vi "Configure Measurement Source.vi"(6 "Measurement Source 2 (0: Channel 1)":i32(ring) items=["Channel 1", "Channel 2", "Channel 3", "Channel 4", "Function 1", "Function 2", "Function 3", "Function 4", "Digital 0", "Digital 1", "Digital 2", "Digital 3", "Digital 4", "Digital 5", "Digital 6", "Digital 7", "Digital 8", "Digital 9", "Digital 10", "Digital 11", "Digital 12", "Digital 13", "Digital 14", "Digital 15", "Memory 1", "Memory 2", "Memory 3", "Memory 4", "Clock", "MTrend", "MSpectrum", "Equalized"], 8 "error in (no error)":errorcluster, 9 "Measurement Source 1 (0: Channel 1)":i32(ring) items=["Channel 1", "Channel 2", "Channel 3", "Channel 4", "Function 1", "Function 2", "Function 3", "Function 4", "Digital 0", "Digital 1", "Digital 2", "Digital 3", "Digital 4", "Digital 5", "Digital 6", "Digital 7", "Digital 8", "Digital 9", "Digital 10", "Digital 11", "Digital 12", "Digital 13", "Digital 14", "Digital 15", "Memory 1", "Memory 2", "Memory 3", "Memory 4", "Clock", "MTrend", "MSpectrum", "Equalized"], 10 "Source Count (0: 1 Source)":u16(ring) items=["1 Source", "2 Source"], 11 "VISA resource name":refnum<visa-resource-name>) -> (0 "error out":errorcluster, 3 "VISA resource name out":refnum<visa-resource-name>)   [LabVIEW 2020, in "Agilent 90000 Series.lvlib"]
doc: "Configures the source for measurements. You can specify one or two sources with this command. Most measurements are made on the first specified source. The delta time measurement uses two sources if two are specified."
uses:
  Agilent 90000 Series.lvlib
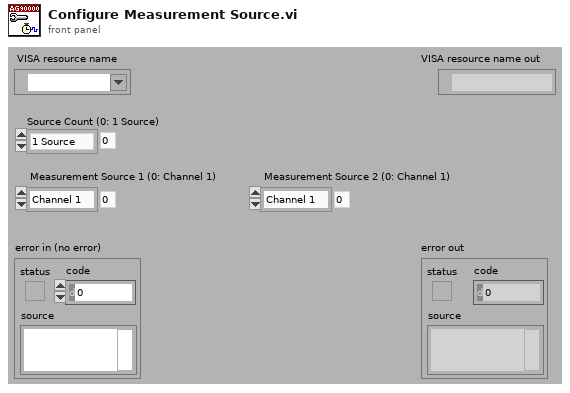
[diagram p1: front panel]
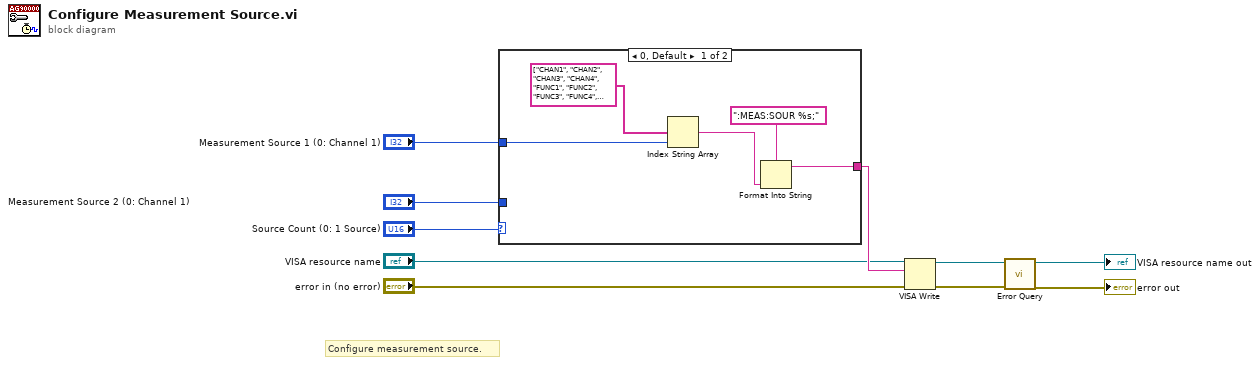
[diagram p0: block diagram]
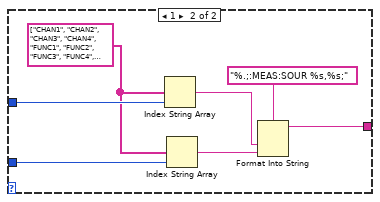
[diagram p2: hidden frame]
diagram:
  # "Configure measurement source."
  n1 = case shown="0, Default" "Source Count (0: 1 Source)" {
    tunnel: "Measurement Source 1 (0: Channel 1)" -> [w14 w22]
    tunnel: [w11 w19] -> w4
    tunnel: "Measurement Source 2 (0: Channel 1)" -> [_ w17]
    frame 0, Default {
      n2 = Index String Array(1:w14, 2:string[] ["CHAN1", "CHAN2", "CHAN3", "CHAN4", "FUNC1", "FUNC2", "FUNC3", "FUNC4", "DIG0", "DIG1", "DIG2", "DIG3", "DIG4", "DIG5", "DIG6", "DIG7", "DIG8", "DIG9", "DIG10", "DIG11", "DIG12", "DIG13", "DIG14", "DIG15", "WMEM1", "WMEM2", "WMEM3", "WMEM4", "CLOC", "MTR", "MSP", "EQU"]) -> (0:w13:string)  [unwired: 1 out]
      n3 = Format Into String(format string=":MEAS:SOUR %s;", w13) -> (resulting string=w11:string)  [unwired: 2 in, 1 out]
    }
    frame 1 {
      w18 = string[] ["CHAN1", "CHAN2", "CHAN3", "CHAN4", "FUNC1", "FUNC2", "FUNC3", "FUNC4", "DIG0", "DIG1", "DIG2", "DIG3", "DIG4", "DIG5", "DIG6", "DIG7", "DIG8", "DIG9", "DIG10", "DIG11", "DIG12", "DIG13", "DIG14", "DIG15", "WMEM1", "WMEM2", "WMEM3", "WMEM4", "CLOC", "MTR", "MSP", "EQU"]
      n4 = Index String Array(1:w22, 2:w18) -> (0:w21:string)  [unwired: 1 out]
      n5 = Index String Array(1:w17, 2:w18) -> (0:w16:string)  [unwired: 1 out]
      n6 = Format Into String(format string="%.;:MEAS:SOUR %s,%s;", w21, w16) -> (resulting string=w19:string)  [unwired: 2 in, 1 out]
    }
  }
  n7 = VISA Write(VISA resource name="VISA resource name", write buffer=w4, error in (no error)="error in (no error)") -> (VISA resource name out=w10:refnum<visa-resource-name>, error out=w9:errorcluster)  [unwired: 1 out]
  n8 = call "Error Query.vi"("error in (no error)"=w9, "VISA resource name"=w10) -> ("error out"=→"error out":errorcluster, "VISA resource name out"=→"VISA resource name out":refnum<visa-resource-name>)  [unwired: 8 out]
